vi "CFG Load Parameters.vi"(0 "Cluster In Ref":refnum<vi>, 5 "Cluster Out Ref":refnum<vi>, 7 "Enum Ref":refnum<vi>, 11 "Error in (no error)":errorcluster, 12 "Keys (Empty:All)":string[](array[string])) -> (4 "Param/Limits":T1[](array[typedef]), 15 "error out":errorcluster)   [LabVIEW 2017]
uses:
  Type Defs/CFG Key Cluster.ctl
  Type Defs/CFG Tag Type Enum.ctl
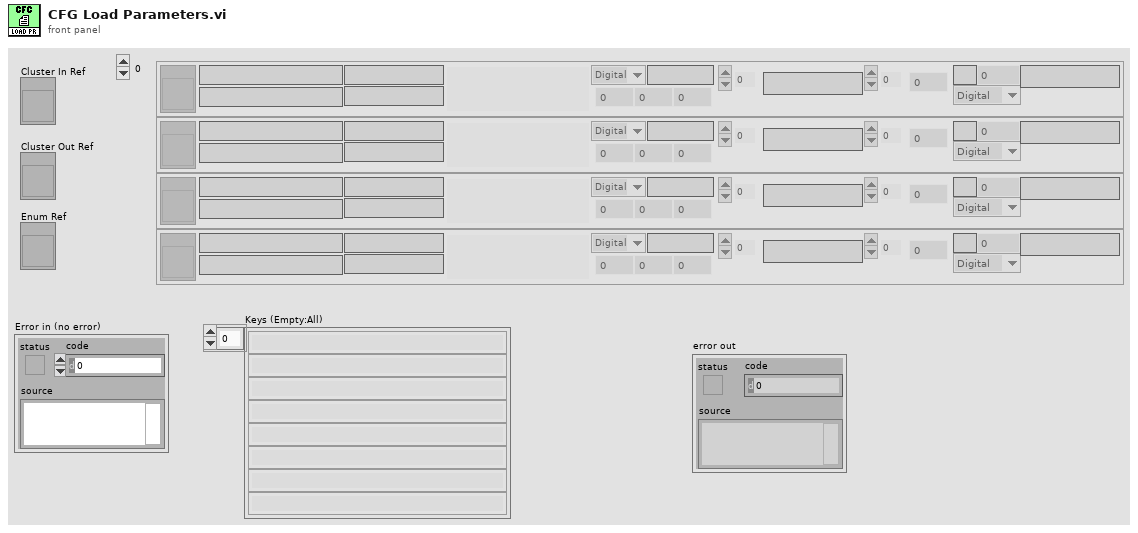
[diagram p1: front panel]
types:
  T1 = typedef "CFG Key Cluster.ctl" = cluster{"Strings []":string[], "Disabled Items []":i32[], "Value":variant, "Format String":string, "Tag":string, "Type":T2, "Section":string, " Ctl Ref":refnum<vi>, "Data Range":cluster{"Minimum":dbl, "Maximum":dbl, "Increment":dbl}, "Unit":string, "Special Instructions":string, "Delimiter(s)":string, "Dimensions":i32, "Element Type":T2, "Array Value String":string}
  T2 = typedef "CFG Tag Type Enum.ctl" = enum16{"Digital", "Slide", "Enum", "Boolean", "String", "Path", "Array", "VISAResourceName", "DAQmxName", "Cluster"}
  T3 = typedef "LVMinMaxIncTypeDef.ctl" = cluster{"Minimum":dbl, "Maximum":dbl, "Increment":dbl}
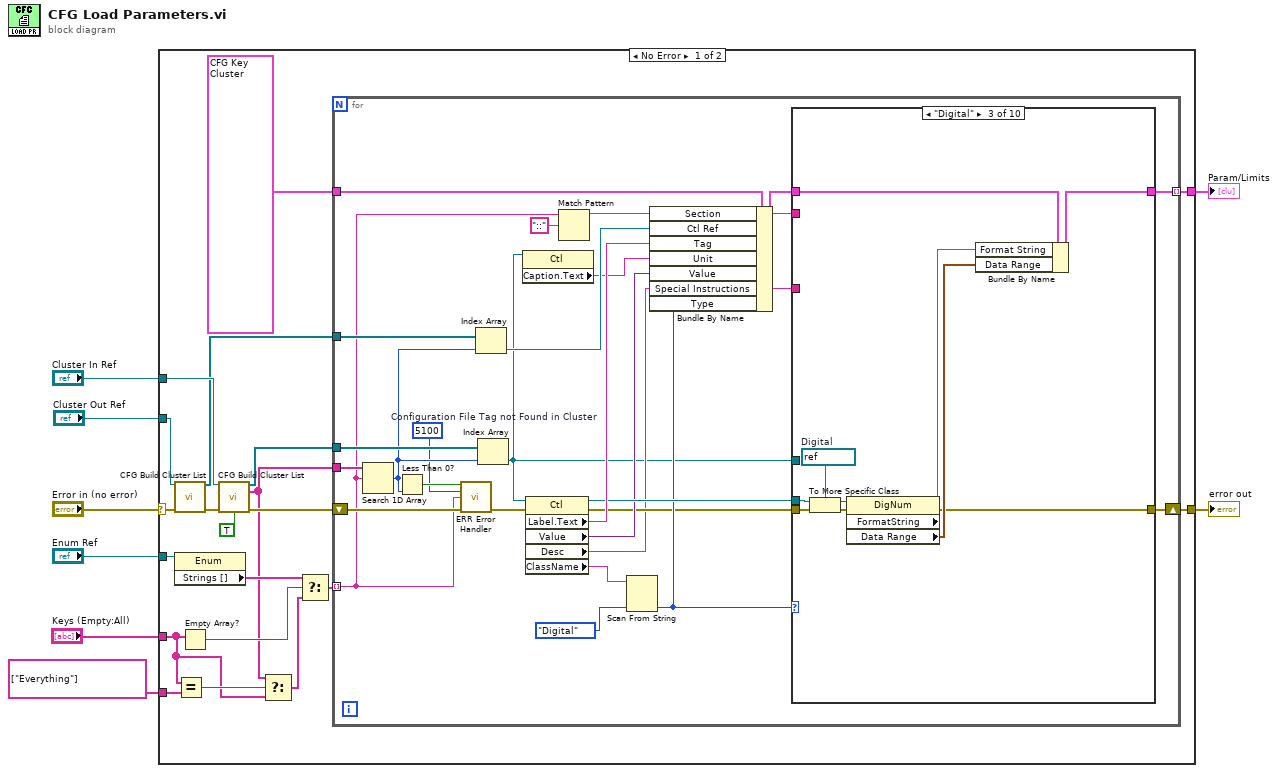
[diagram p0: block diagram]
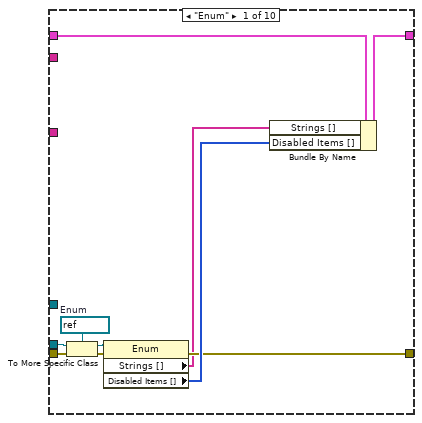
[diagram p2: hidden frame]
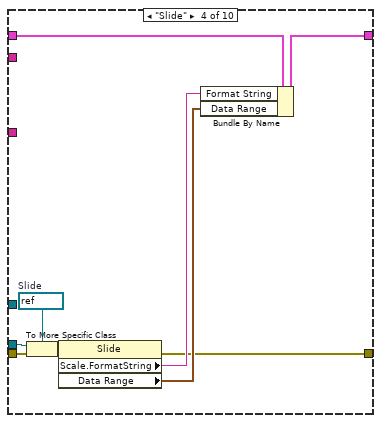
[diagram p4: hidden frame]
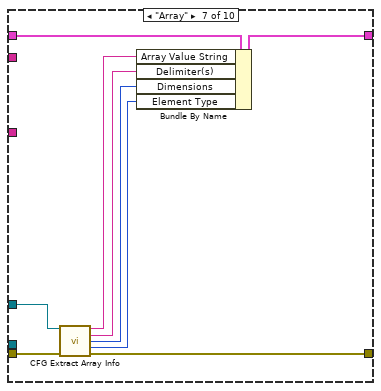
[diagram p7: hidden frame]
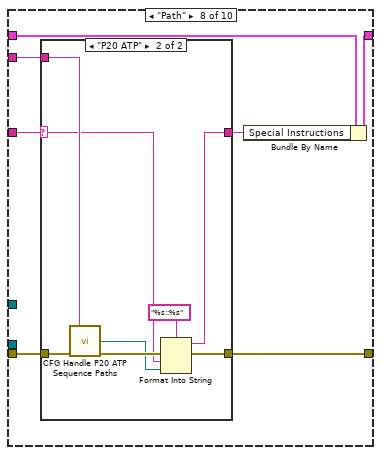
[diagram p8: hidden frame]
diagram:
  n1 = case shown="No Error" "Error in (no error)" {
    selector: "Error in (no error)" -> [w21 w121]
    tunnel: [w27 _] -> w8
    tunnel: [w26 w121] -> w6
    tunnel: "Cluster In Ref" -> [w23 _]
    tunnel: "Enum Ref" -> [w25 _]
    tunnel: "Cluster Out Ref" -> [w19 _]
    tunnel: "Keys (Empty:All)" -> [w10 _]
    tunnel: string[] ["Everything"] ("Keys (Empty:All)") -> [w13 _]
    frame No Error {
      n2 = call "CFG Build Cluster List.vi"("Cluser Ref"=w19, "Error in (no error)"=w21) -> ("Item Refs"=w18:refnum<vi>[], "error out"=w20:errorcluster)  [unwired: 1 in, 11 out]
      n3 = property class="Enum"(reference=w25) -> ("Strings []"=w17:string[])  [unwired: 1 in, 2 out]
      n4 = Equal?(x=w10, y=w13) -> (x = y?=w11:bool)
      n5 = Empty Array?(array=w10) -> (empty?=w16:bool)
      n6 = call "CFG Build Cluster List.vi"("Cluser Ref"=w23, "Error in (no error)"=w20, "Build Item Names (F)"=TRUE) -> ("Item Refs"=w22:refnum<vi>[], "Item Names"=w12:string[], "error out"=w24:errorcluster)  [unwired: 10 out]
      n7 = Select(t=w12, s=w11, f=w10) -> (s? t:f=w9:string[])
      n8 = Select(t=w17, s=w16, f=w9) -> (s? t:f=w15:string[])
      n9 = for {
        tunnel: w15 -> [w35] mode=indexing
        tunnel: T1 {"Strings []"=[], "Disabled Items []"=[], "Value"=variant, "Format String"="", "Tag"="", "Type"=enum."Digital", "Section"="", " Ctl Ref"=refnum, "Data Range"={"Minimum"=0.0, "Maximum"=0.0, "Increment"=0.0}, "Unit"="", "Special Instructions"="", "Delimiter(s)"="", "Dimensions"=0, "Element Type"=enum."Digital", "Array Value String"=""} ("Tag Cluster") -> [w53]
        shift-right: [w49] -> w26
        shift-left: w24 -> [w39]
        tunnel: [w46] -> w27 mode=indexing
        tunnel: w12 -> [w51]
        tunnel: w22 -> [w50]
        tunnel: w18 -> [w41]
        w36 = 5100  # Configuration File Tag not Found in Cluster
        n10 = Search 1D Array(1D array=w51, element=w35) -> (index of element=w38:i32)  [unwired: 1 out]
        n11 = Less Than 0?(x=w38) -> (x < 0?=w37:bool)
        n12 = call "ERR Error Handler.vi"("Error Status"=w37, "Error Code"=w36, "Cause Of Error"=w35, "Error In (no error)"=w39) -> ("Error Out"=w34:errorcluster)  [unwired: 2 in, 9 out]
        n13 = Index Array(array=w41, index=w38) -> (element=w40:refnum<vi>)
        n14 = Index Array(array=w50, index=w38) -> (element=w29:refnum<vi>)
        n15 = property class="Ctl"(reference=w29) -> ("Caption.Text"=w32:string)  [unwired: 1 in, 2 out]
        n16 = property class="Ctl"(reference=w29, error in=w34) -> (reference out=w48:refnum<vi>, error out=w33:errorcluster, "Label.Text"=w52:string, "Value"=w44:variant, "Desc"=w30:string, "ClassName"=w43:string)
        n17 = Match Pattern(string=w35, regular expression="::") -> (before substring=w31:string)  [unwired: 4 out]
        n18 = Scan From String(input string=w43, default 1=CFG_Tag_Type_Enum."Digital" ("Type")) -> (output 1=w42:T2)  [unwired: 3 in, 3 out]
        n19 = Bundle By Name(cluster=w53, "Section"=w31, "Ctl Ref"=w40, "Tag"=w52, "Unit"=w32, "Value"=w44, "Special Instructions"=w30, "Type"=w42) -> (w47:T1)
        n20 = case shown="\"Digital\"" w42 {
          tunnel: w48 -> [w63 _ w75 w85 _ _ _ _ _ _]
          tunnel: w47 -> [w61 w65 w73 w83 w88 w90 w96 w102 w118 w120]
          tunnel: [w59 w65 w72 w82 w88 w90 w95 w101 w118 w120] -> w46
          tunnel: w33 -> [w58 w66 w70 w80 w87 w89 w99 w106 w117 w119]
          tunnel: [w56 w66 w67 w77 w87 w89 w98 w104 w117 w119] -> w49
          tunnel: w31 -> [_ _ _ _ _ _ _ w105 _ _]
          tunnel: w30 -> [_ _ _ _ _ _ _ w100 _ _]
          tunnel: w29 -> [_ _ _ _ _ _ w97 _ _ _]
          frame "Enum" {
            w64 = refnum<vi> refnum  # Enum
            n21 = To More Specific Class(target class=w64, reference=w63, error in=w58) -> (specific class reference=w62:refnum<vi>, error out=w57:errorcluster)
            n22 = property class="Enum"(reference=w62, error in=w57) -> (error out=w56:errorcluster, "Strings []"=w55:string[], "Disabled Items []"=w60:i32[])  [unwired: 1 out]
            n23 = Bundle By Name(cluster=w61, "Strings []"=w55, "Disabled Items []"=w60) -> (w59:T1)
          }
          frame "Cluster" {
          }
          frame "Digital" {
            w76 = refnum<vi> refnum  # Digital
            n24 = To More Specific Class(target class=w76, reference=w75, error in=w70) -> (specific class reference=w69:refnum<vi>, error out=w74:errorcluster)
            n25 = property class="DigNum"(reference=w69, error in=w74) -> (error out=w67:errorcluster, "FormatString"=w68:string, "Data Range"=w71:T3)  [unwired: 1 out]
            n26 = Bundle By Name(cluster=w73, "Format String"=w68, "Data Range"=w71) -> (w72:T1)
          }
          frame "Slide" {
            w86 = refnum<vi> refnum  # Slide
            n27 = To More Specific Class(target class=w86, reference=w85, error in=w80) -> (specific class reference=w79:refnum<vi>, error out=w84:errorcluster)
            n28 = property class="Slide"(reference=w79, error in=w84) -> (error out=w77:errorcluster, "Scale.FormatString"=w78:string, "Data Range"=w81:T3)  [unwired: 1 out]
            n29 = Bundle By Name(cluster=w83, "Format String"=w78, "Data Range"=w81) -> (w82:T1)
          }
          frame "Boolean" {
          }
          frame "String" {
          }
          frame "Array" {
            n30 = call "CFG Extract Array Info.vi"("reference"=w97, "error in"=w99) -> ("Value String"=w94:string, "Delimiter(s)"=w93:string, "Dimensions"=w92:i32, "Element Type"=w91:T2, "error out"=w98:errorcluster)  [unwired: 9 out]
            n31 = Bundle By Name(cluster=w96, "Array Value String"=w94, "Delimiter(s)"=w93, "Dimensions"=w92, "Element Type"=w91) -> (w95:T1)
          }
          frame "Path" {
            n32 = case shown="\"P20 ATP\"" w100 {
              selector: w100 -> [w108 w109]
              tunnel: w106 -> [w107 w116]
              tunnel: w105 -> [_ w115]
              tunnel: [w107 w113] -> w104
              tunnel: [w108 w110] -> w103
              frame Default {
              }
              frame "P20 ATP" {
                n33 = call "CFG Handle P20 ATP Sequence Paths.vi"("Section"=w115, "Error In (no error)"=w116) -> ("Start Path"=w112:path, "error out"=w114:errorcluster)  [unwired: 1 in, 11 out]
                n34 = Format Into String(format string="%s::%s", error in=w114, w109, w112) -> (resulting string=w110:string, error out=w113:errorcluster)  [unwired: 1 in]
              }
            }
            n35 = Bundle By Name(cluster=w102, "Special Instructions"=w103) -> (w101:T1)
          }
          frame "VISAResourceName" {
          }
          frame "DAQmxName" {
          }
        }
      }
    }
    frame Error {
    }
  }
  "Param/Limits" <- w8
  "error out" <- w6
